vi "OC2 create report array.vi"(3 "error in":errorcluster, 4 "report string":string, 5 "rx packet ok":bool=TRUE) -> (0 "Report cluster":T1 {"Checksum" format="%x"}, 1 "error out":errorcluster)   [LabVIEW 2009]
panel:
  # "Create report array"
  # "j520.004;0.002;4;4;100.151;100.151;100.000;100.000;1;1;16"
  # "V1.02"
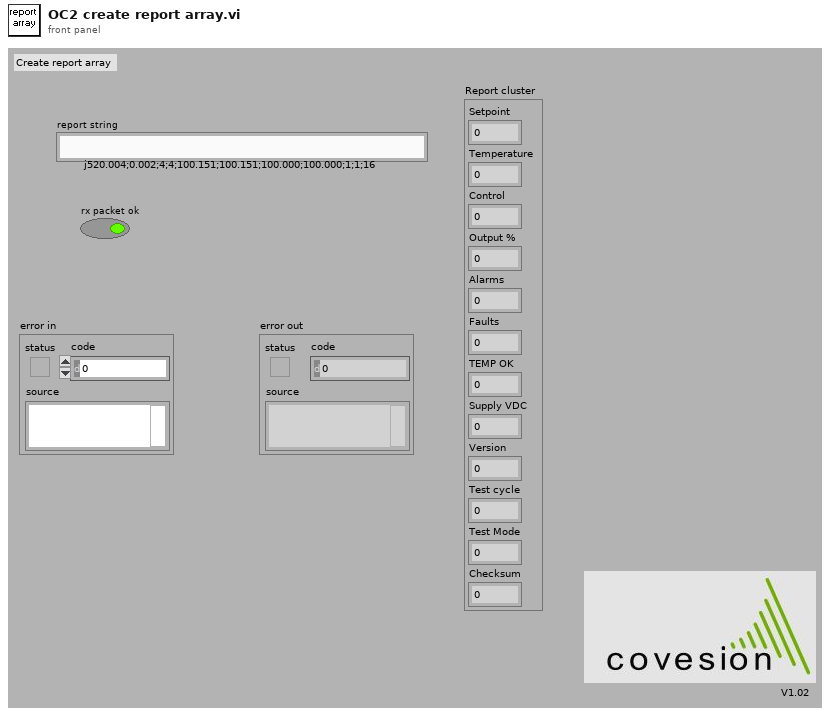
[diagram p1: front panel]
types:
  T1 = cluster{"Setpoint":dbl, "Temperature":dbl, "Control":i32, "Output %":dbl, "Alarms":i32, "Faults":i32, "TEMP OK":i32, "Supply VDC":dbl, "Version":dbl, "Test cycle":i32, "Test Mode":i32, "Checksum":i32}
  T2 = cluster{dbl, dbl, i32, dbl, i32, i32, i32, dbl, dbl, i32, i32, i32}
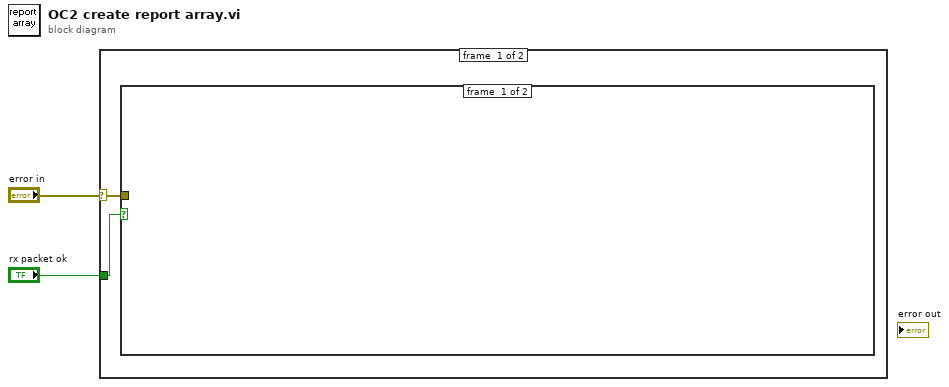
[diagram p0: block diagram]
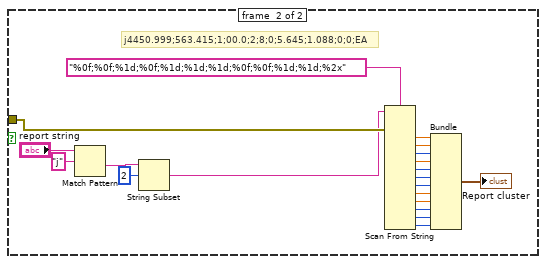
[diagram p2: hidden frame]
diagram:
  n1 = case shown="No Error" "error in" {
    selector: "error in" -> [w4 _]
    tunnel: "rx packet ok" -> [w3 _]
    frame #0 {
      n2 = case shown="True" w3 {
        tunnel: w4 -> [_ w24]
        frame #0 {
        }
        frame #1 {
          # "j4450.999;563.415;1;00.0;2;8;0;5.645;1.088;0;0;EA"
          n3 = Match Pattern(string="report string", regular expression="j") -> (after substring=w20:string)  [unwired: 1 in, 3 out]
          n4 = String Subset(string=w20, offset (0)=u32 2 ("initial scan location")) -> (substring=w19:string)  [unwired: 1 in]
          n5 = Scan From String(format string="%0f;%0f;%1d;%0f;%1d;%1d;%1d;%0f;%0f;%1d;%1d;%2x" ("regular expression"), input string=w19, error in=w24) -> (output 1=w18:dbl, output 2=w17:dbl, output 3=w16:i32, output 4=w15:dbl, output 5=w14:i32, output 6=w13:i32, output 7=w12:i32, output 8=w11:dbl, output 9=w10:dbl, output 10=w9:i32, output 11=w8:i32, output 12=w6:i32)  [unwired: 13 in, 3 out]
          n6 = Bundle(w18, w17, w16, w15, w14, w13, w12, w11, w10, w9, w8, w6) -> (→"Report cluster":T2)  [unwired: 1 in]
        }
      }
    }
    frame #1 {
    }
  }
